vi "Proyecto Interciclo Autotronica_Espinoza_Moreno_Morales_Pualasin.vi"() -> ()   [LabVIEW 2025]
uses:
  <vilib>/MakerHub/LINX/Private/Type Defs/LINX Ref.ctl
  <vilib>/MakerHub/LINX/Private/Type Defs/Platform.ctl
  <vilib>/MakerHub/LINX/Private/Type Defs/Interface.ctl
  <vilib>/MakerHub/LINX/Private/Device/Type Defs/LINX Device Config.ctl
  <vilib>/MakerHub/LINX/Private/Device/Type Defs/TCP Config.ctl
  <vilib>/MakerHub/LINX/Private/Device/Type Defs/Channels.ctl
  <vilib>/MakerHub/LINX/Public/Peripherals/Digital/Digital Read 1 Chan.vi
  <vilib>/MakerHub/LINX/Public/Peripherals/Analog/Analog Read 1 Chan.vi
  <vilib>/MakerHub/LINX/Public/Peripherals/Digital/Digital Read N Chans.vi
  <vilib>/MakerHub/LINX/Public/Peripherals/Analog/Analog Read N Chans.vi
  <vilib>/MakerHub/LINX/Private/Local IO/LinxDigitalRead.vi
  <vilib>/MakerHub/LINX/Public/Utilities/Check Channel.vi
  <vilib>/MakerHub/LINX/Private/Local IO/LinxAnalogRead.vi
  <vilib>/MakerHub/LINX/Public/Utilities/Open Serial.vi
  <vilib>/MakerHub/LINX/Private/Utilties/Generate Error.vi
  <vilib>/express/express shared/transition.llb/Dynamic To Waveform Array.vi
  <vilib>/express/express signal manip/GetorSetDDTAttributes/Set DDT Attributes/SetT0.vi
  <vilib>/express/express shared/transition.llb/Waveform Array To Dynamic.vi
  <vilib>/express/express signal manip/GetorSetDDTAttributes/Set DDT Attributes/Set DDT Properties.xnode
  <vilib>/express/express arith-compare/Formula/XNode/ExpressFormulaBlockNode.xnode
  <vilib>/MakerHub/LINX/LMH-LINX.lvlib
  <vilib>/MakerHub/LINX/Private/Device/Device.lvlib
panel:
  in  "Stop":bool
  out "Kelvin":dbl(slide) scale=250.0..400.0
  out "Fahrenheit":dbl(slide) scale=0.0..220.0
  out "CARGA DE BATERIA":dbl(knob) scale=0.0..100.0
  out "PRESION DE FRENADO":dbl(graph)
  out "PRESION DE NEUMATICOS PSI":dbl(knob) scale=0.0..40.0
  out "TEMPERATURA AMBIENTE":dbl(slide) scale=0.0..100.0
  in  "Serial Port":refnum<visa-resource-name>="N/A"
  # "Fahrenheit"
  # "Kelvin"
  # "TEMPERATURA AMBIENTE"
  # "PRESION DE FRENADO"
  # "CARGA DE BATERIA"
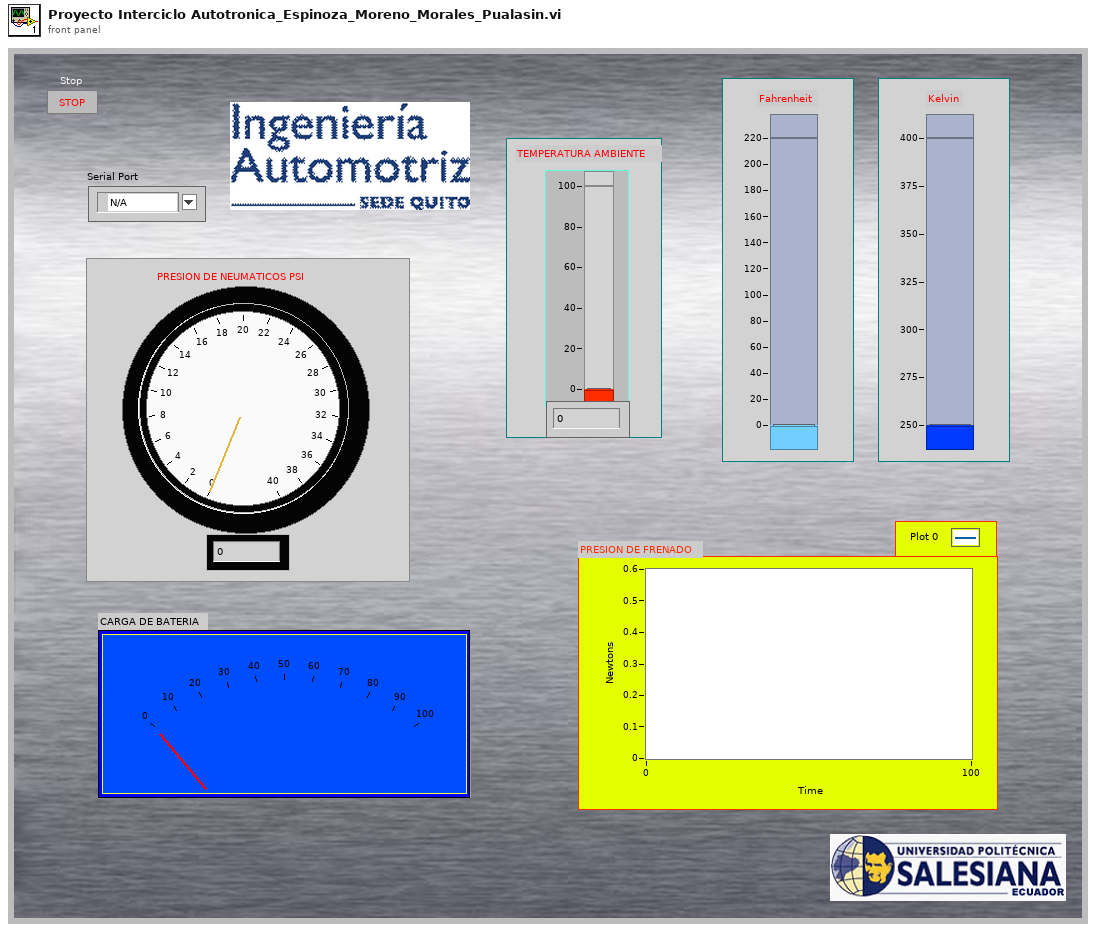
[diagram p1: front panel]
types:
  T1 = typedef "LMH-LINX.lvlib/LINX Ref.ctl" = cluster{"IO":T2, "Interface":T3, "LINX Device Config":T4}
  T2 = typedef "LMH-LINX.lvlib/Platform.ctl" = enum16{"Remote", "Local"}
  T3 = typedef "LMH-LINX.lvlib/Interface.ctl" = enum16{"Serial", "TCP"}
  T4 = typedef "LMH-LINX.lvlib/Device.lvlib/LINX Device Config.ctl" = cluster{"Interface":T3, "COM Port":refnum<visa-resource-name>, "TCP Configuration":T5, "Device Family":u8, "Device ID":u8, "Device Name":string, "TCP Ref":refnum<k5>, "Channels":T6}
  T5 = typedef "LMH-LINX.lvlib/Device.lvlib/TCP Config.ctl" = cluster{"IP Address":string, "Port":u16}
  T6 = typedef "LMH-LINX.lvlib/Channels.ctl" = cluster{"DI":u8[], "DO":u8[], "AI":u8[], "AO":u8[], "PWM":u8[], "QE":u8[], "UART":u8[], "I2C 2":u8[], "SPI":u8[], "CAN":u8[], "Servo":u8[], "AI Ref (V)":dbl, "AI Resolution (Bits)":u8, "AO Ref (V)":dbl, "AO Resolution (Bits)":u8}
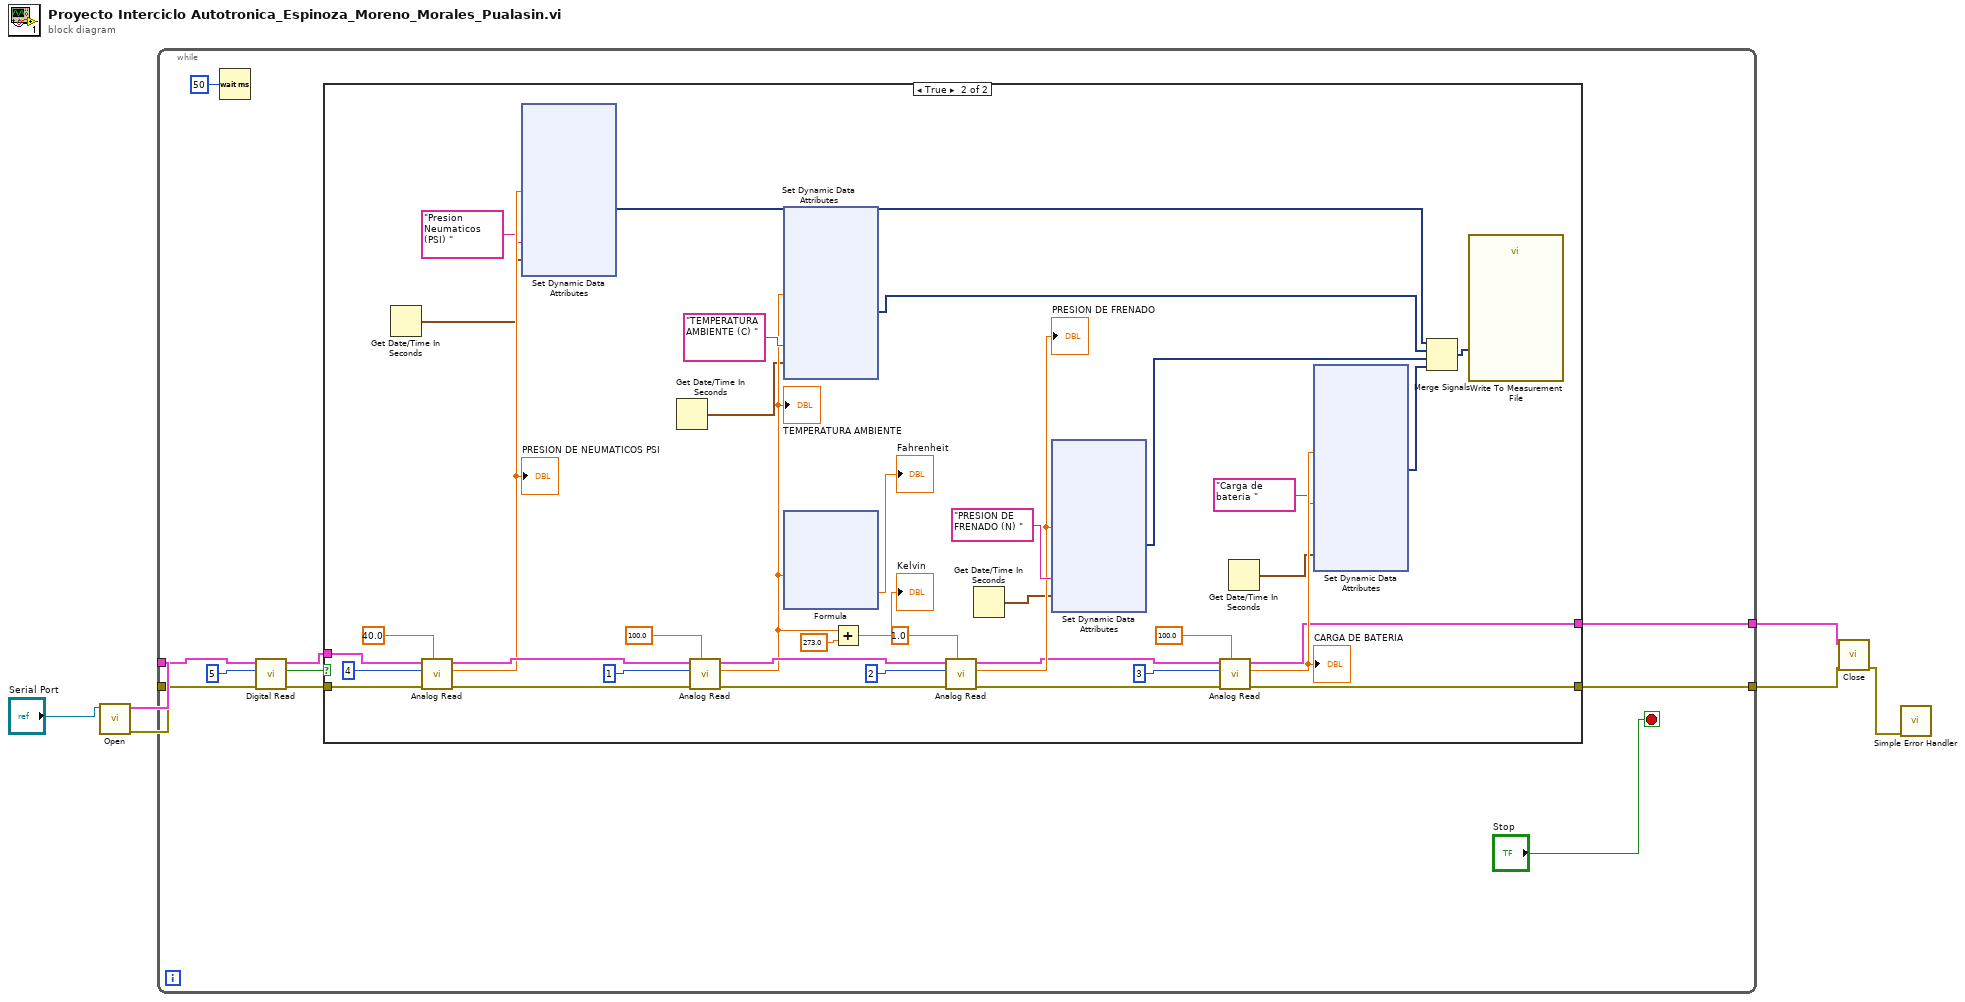
[diagram p0: block diagram]
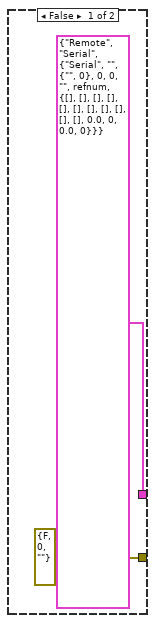
[diagram p2: hidden frame]
diagram:
  n1 = call-poly <vilib>:"Open.vi"("Serial Port"="Serial Port") -> ("Error Out"=w4:errorcluster, "LINX Resource"=w6:T1)  [unwired: 8 in, 1 out]
  n2 = while {
    tunnel: w6 -> [w15]
    tunnel: [w9] -> w5
    tunnel: w4 -> [w14]
    tunnel: [w8] -> w3
    stop <- "Stop" stop-if-true
    n3 = Wait (ms)(milliseconds to wait=u32 50) -> ()  [unwired: 1 out]
    n4 = call-poly <vilib>:"Digital Read.vi"("Error In"=w14, "DI Channel"=u8 5, "LINX Resource"=w15) -> ("Error Out"=w10:errorcluster, "DI Value"=w12:bool, "LINX Resource"=w11:T1)  [unwired: 6 in]
    n5 = case shown="True" w12 {
      tunnel: w11 -> [_ w26]
      tunnel: w10 -> [_ w25]
      tunnel: [T1 {"IO"=enum."Remote", "Interface"=enum."Serial", "LINX Device Config"={"Interface"=enum."Serial", "COM Port"="", "TCP Configuration"={"IP Address"="", "Port"=0}, "Device Family"=0, "Device ID"=0, "Device Name"="", "TCP Ref"=refnum, "Channels"={"DI"=[], "DO"=[], "AI"=[], "AO"=[], "PWM"=[], "QE"=[], "UART"=[], "I2C 2"=[], "SPI"=[], "CAN"=[], "Servo"=[], "AI Ref (V)"=0.0, "AI Resolution (Bits)"=0, "AO Ref (V)"=0.0, "AO Resolution (Bits)"=0}}} ("LINX Resource") w24] -> w9
      tunnel: [errorcluster {"status"=FALSE, "code"=0, "source"=""} ("Error Out") w23] -> w8
      frame False {
      }
      frame True {
        n6 = Get Date/Time In Seconds() -> (seconds since 1Jan1904=w19:timestamp)
        n7 = call-poly <vilib>:"Analog Read.vi"("Analog Ref Override (V)"=40.0, "Error In"=w25, "Analog Channel"=u8 4, "LINX Resource"=w26) -> ("Error Out"=w54:errorcluster, "Voltage"=w45:dbl, "LINX Resource"=w56:T1)  [unwired: 4 in, 1 out]
        "PRESION DE NEUMATICOS PSI" <- w45
        n8 = xnode "Set Dynamic Data Attributes"("Signals In"=w45, "Signal Name"="Presion Neumaticos (PSI) ", "Timestamp"=w19) -> ("Signals Out"=w41:dynamicdata)  [unwired: 2 in, 1 out]
        n9 = Get Date/Time In Seconds() -> (seconds since 1Jan1904=w20:timestamp)
        n10 = call-poly <vilib>:"Analog Read.vi"("Analog Ref Override (V)"=100.0, "Error In"=w54, "Analog Channel"=u8 1, "LINX Resource"=w56) -> ("Error Out"=w53:errorcluster, "Voltage"=w37:dbl, "LINX Resource"=w55:T1)  [unwired: 4 in, 1 out]
        "TEMPERATURA AMBIENTE" <- w37
        n11 = xnode "Set Dynamic Data Attributes"("Signals In"=w37, "Signal Name"="TEMPERATURA AMBIENTE (C) ", "Timestamp"=w20) -> ("Signals Out"=w40:dynamicdata)  [unwired: 2 in, 1 out]
        n12 = xnode "Formula"("X1"=w37) -> ("Result"=→"Fahrenheit":dbl)  [unwired: 1 in, 1 out]
        n13 = Add(x=w37, y=273.0 ("Kelvin")) -> (x+y=→"Kelvin":dbl)
        n14 = call-poly <vilib>:"Analog Read.vi"("Analog Ref Override (V)"=1.0, "Error In"=w53, "Analog Channel"=u8 2, "LINX Resource"=w55) -> ("Error Out"=w33:errorcluster, "Voltage"=w39:dbl, "LINX Resource"=w32:T1)  [unwired: 4 in, 1 out]
        "PRESION DE FRENADO" <- w39
        n15 = Get Date/Time In Seconds() -> (seconds since 1Jan1904=w21:timestamp)
        n16 = xnode "Set Dynamic Data Attributes"("Signals In"=w39, "Signal Name"="PRESION DE FRENADO (N) ", "Timestamp"=w21) -> ("Signals Out"=w38:dynamicdata)  [unwired: 2 in, 1 out]
        n17 = call-poly <vilib>:"Analog Read.vi"("Analog Ref Override (V)"=100.0, "Error In"=w33, "Analog Channel"=u8 3, "LINX Resource"=w32) -> ("Error Out"=w23:errorcluster, "Voltage"=w29:dbl, "LINX Resource"=w24:T1)  [unwired: 4 in, 1 out]
        "CARGA DE BATERIA" <- w29
        n18 = Get Date/Time In Seconds() -> (seconds since 1Jan1904=w22:timestamp)
        n19 = xnode "Set Dynamic Data Attributes"("Signals In"=w29, "Signal Name"="Carga de bateria ", "Timestamp"=w22) -> ("Signals Out"=w27:dynamicdata)  [unwired: 2 in, 1 out]
        n20 = Merge Signals(w41, w40, w38, w27) -> (w46:dynamicdata)
        n21 = call "Write To Measurement File"("Signals"=w46) -> ()  [unwired: 16 in, 3 out]
      }
    }
  }
  n22 = call <vilib>:"Close.vi"("Error In"=w3, "LINX Resource"=w5) -> ("Error Out"=w2:errorcluster)  [unwired: 9 in]
  n23 = call <vilib>:"Simple Error Handler.vi"("error in (no error)"=w2) -> ()  [unwired: 4 in, 5 out]
